vi "恢复参数.vi"(8 "仪器公式":T1(array[cluster]), 9 "量程参数":T2(array[cluster]), 10 "试剂容量参数":T3, 11 "外设参数":cluster{"外设配置":T4, "error out":errorcluster} {"外设配置"."阀方向" items=["顺时针", "逆时针", "就近"]; "外设配置"."总氮x公式0" items=["0", "1"]; "外设配置"."光谱仪类型" items=["1型", "2型", "3型", "2型氙灯联控"]; "外设配置"."泵阀量" items=["9通"=9, "10通"=10, "12通"=12]; "外设配置"."泵类型" items=["1型", "2型", "sy04型+旋转阀"]}) -> (3 "恢复结果":string)   [LabVIEW 2016, in "斯坦道氨氮.lvlib"]
uses:
  <vilib>/NI/Progress Bar/Progress Bar.lvlib
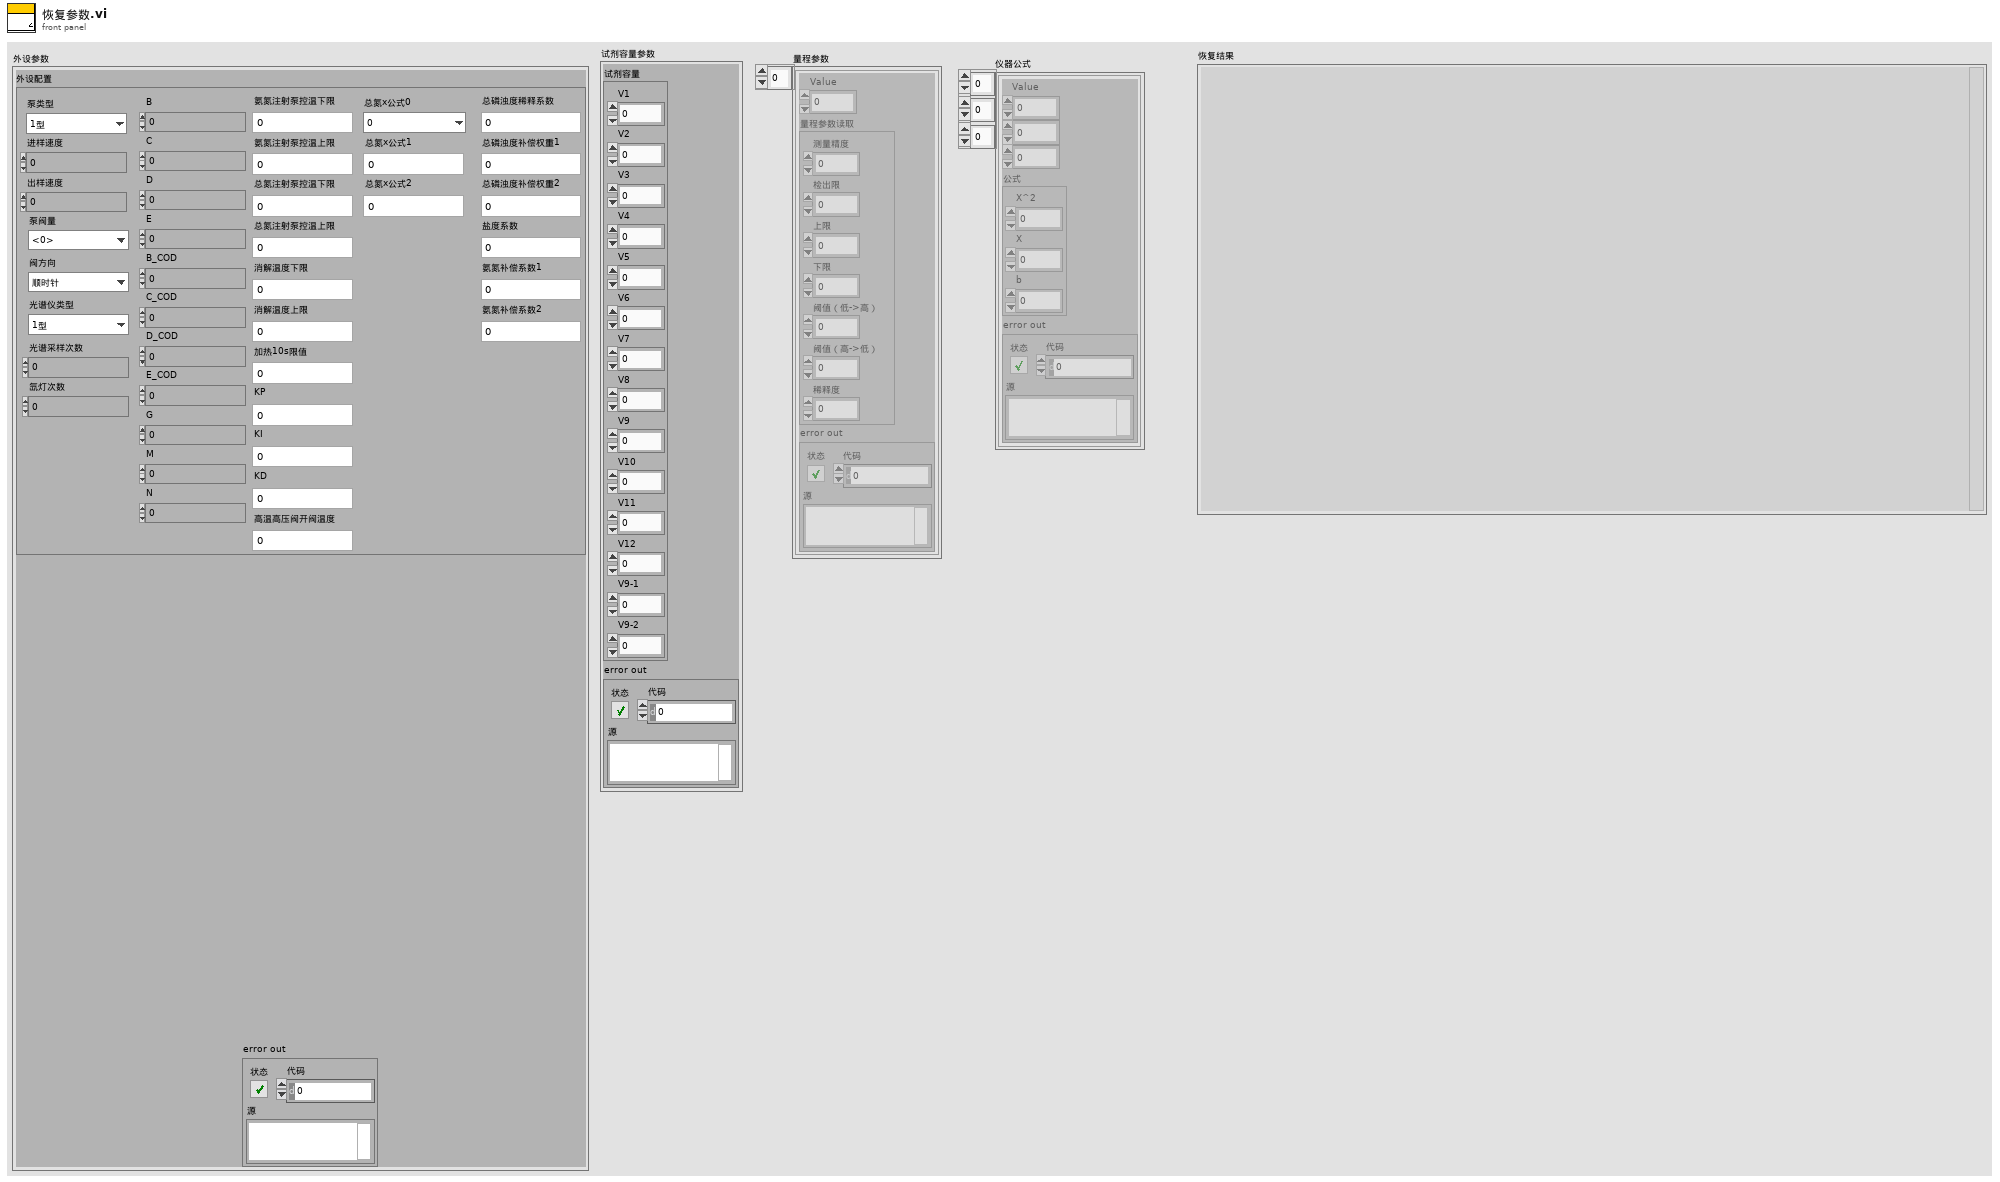
[diagram p1: front panel]
types:
  T1 = cluster{"Value":u16, i32, i32, "公式":cluster{"X^2":dbl, "X":dbl, "b":dbl}, "error out":errorcluster}[][][]
  T2 = cluster{"Value":u16, "量程参数读取":cluster{"测量精度":u16, "检出限":dbl, "上限":dbl, "下限":dbl, "阈值（低->高）":dbl, "阈值（高->低）":dbl, "稀释度":dbl}, "error out":errorcluster}[]
  T3 = cluster{"试剂容量":cluster{"V1":sgl, "V2":sgl, "V3":sgl, "V4":sgl, "V5":sgl, "V6":sgl, "V7":sgl, "V8":sgl, "V9":sgl, "V10":sgl, "V11":sgl, "V12":sgl, "V9-1":sgl, "V9-2":sgl}, "error out":errorcluster}
  T4 = typedef "斯坦道氨氮.lvlib/V3 A版外设参数.ctl" = cluster{"泵类型":u8, "进样速度":u32, "出样速度":u32, "泵阀量":u8, "阀方向":u8, "光谱仪类型":u8, "光谱采样次数":u8, "氙灯次数":u8, "B":u16, "C":u16, "D":u16, "E":u16, "B_COD":u16, "C_COD":u16, "D_COD":u16, "E_COD":u16, "G":u16, "M":u16, "N":u16, "氨氮注射泵控温下限":sgl, "氨氮注射泵控温上限":sgl, "总氮注射泵控温下限":sgl, "总氮注射泵控温上限":sgl, "消解温度下限":sgl, "消解温度上限":sgl, "加热10s限值":sgl, "KP":sgl, "KI":sgl, "KD":sgl, "高温高压阀开阀温度":sgl, "总氮x公式0":u8, "总氮x公式1":sgl, "总氮x公式2":sgl, "总磷浊度稀释系数":sgl, "总磷浊度补偿权重1":sgl, "总磷浊度补偿权重2":sgl, "盐度系数":sgl, "氨氮补偿系数1":sgl, "氨氮补偿系数2":sgl}
  T5 = enum16{"恢复外设参数", "恢复试剂容量参数", "恢复量程参数", "恢复仪器公式", "结束"}
  T6 = cluster{"V1":sgl, "V2":sgl, "V3":sgl, "V4":sgl, "V5":sgl, "V6":sgl, "V7":sgl, "V8":sgl, "V9":sgl, "V10":sgl, "V11":sgl, "V12":sgl, "V9-1":sgl, "V9-2":sgl}
  T7 = cluster{"测量精度":u16, "检出限":dbl, "上限":dbl, "下限":dbl, "阈值（低->高）":dbl, "阈值（高->低）":dbl, "稀释度":dbl}
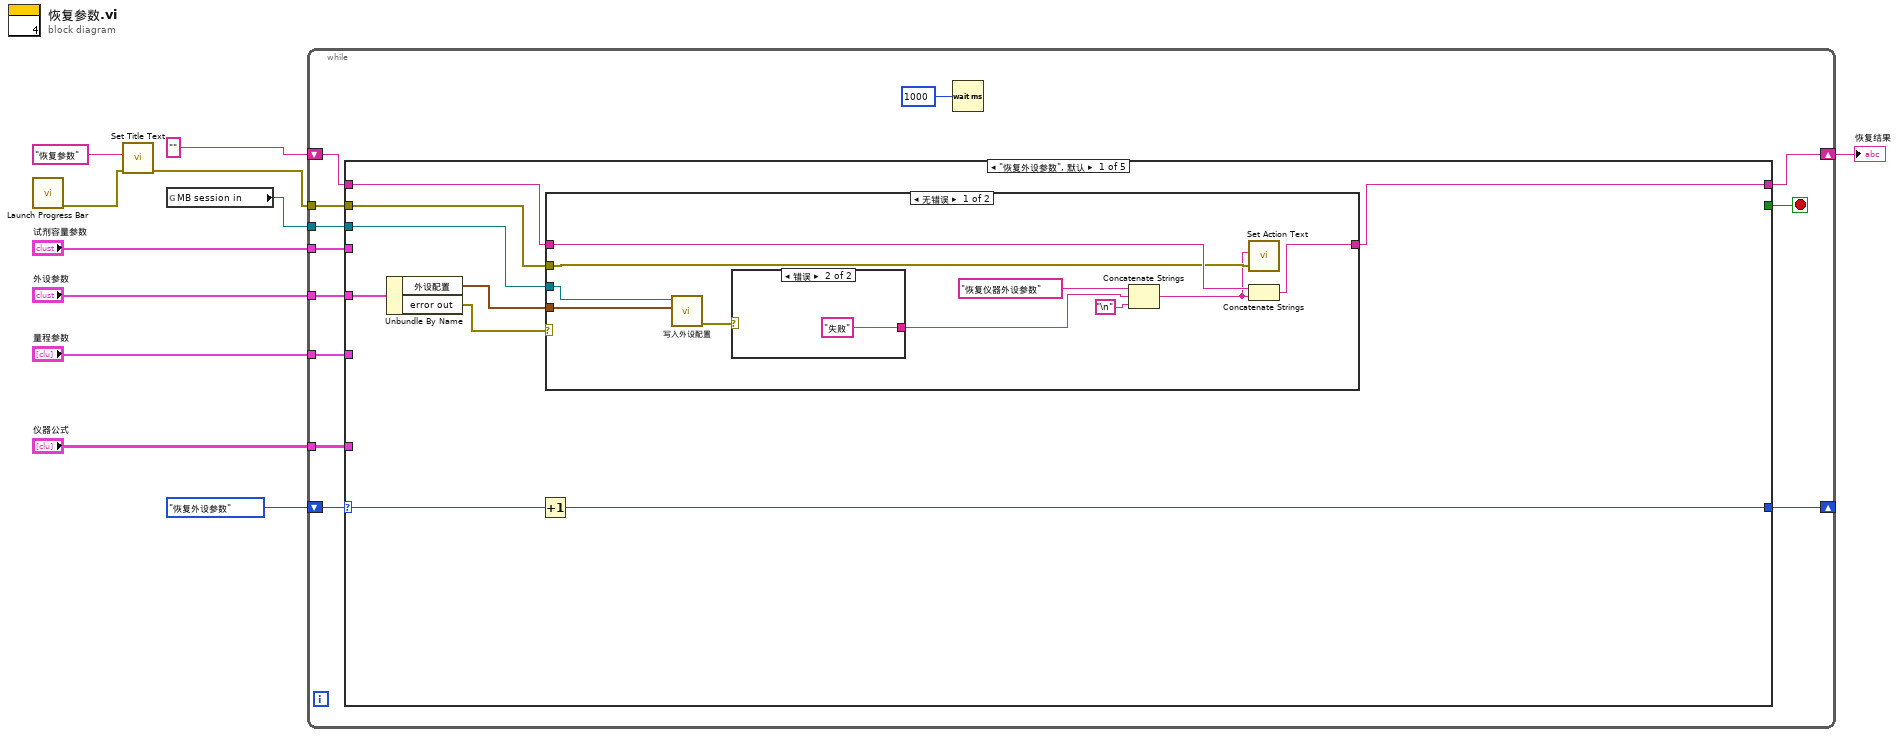
[diagram p0: block diagram]
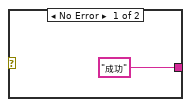
[diagram p2: hidden frame]
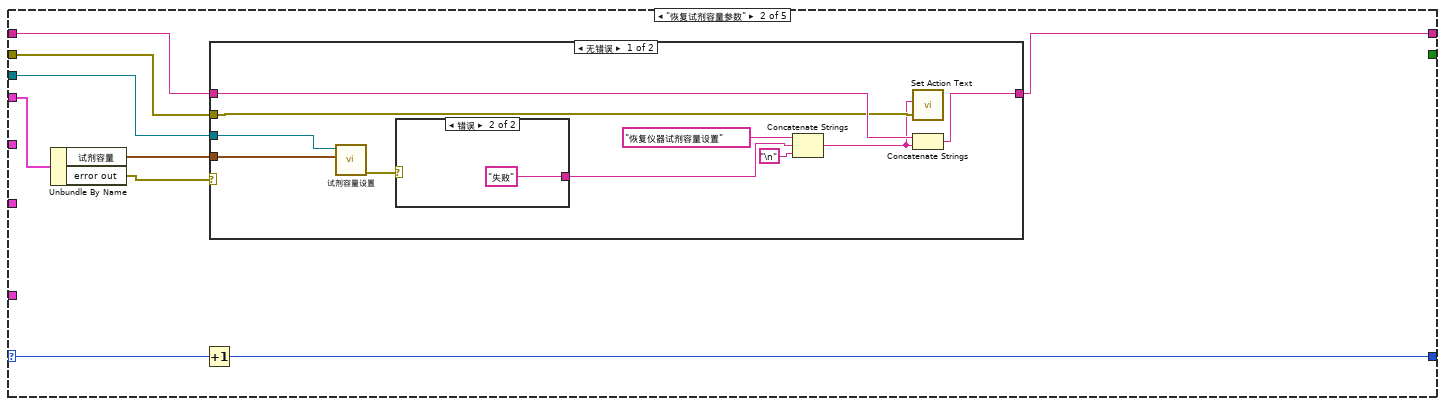
[diagram p4: hidden frame]
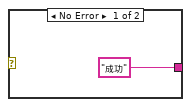
[diagram p5: hidden frame]
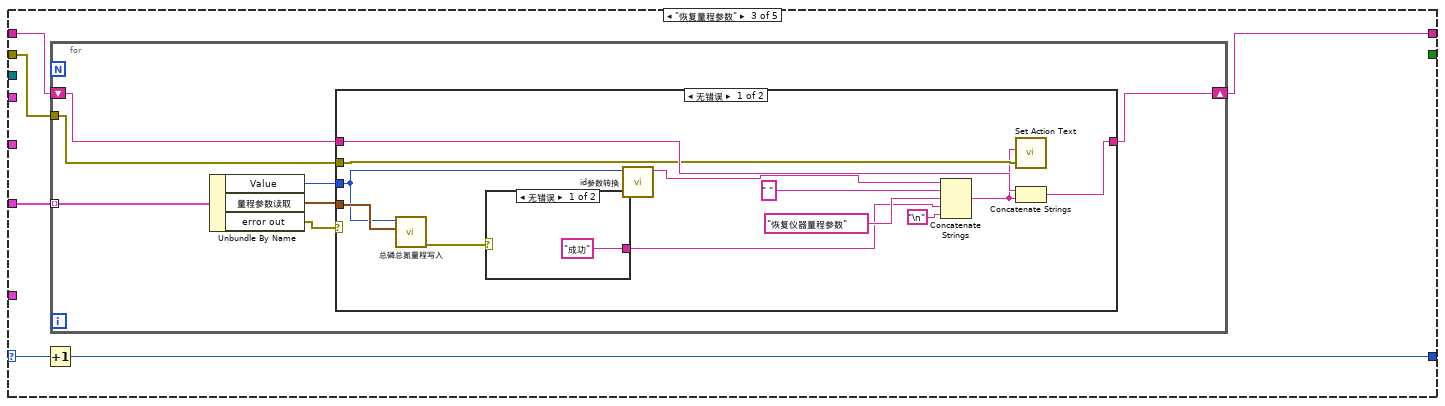
[diagram p7: hidden frame]
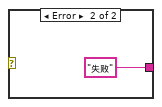
[diagram p8: hidden frame]
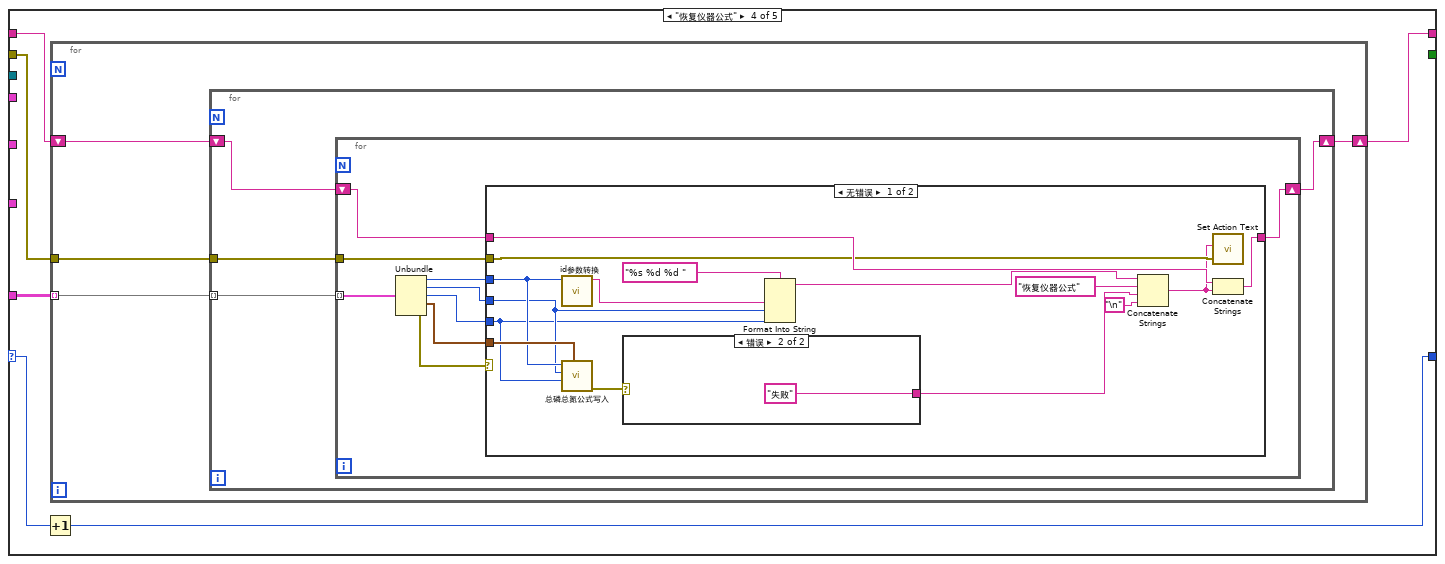
[diagram p10: hidden frame]
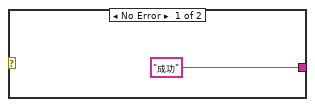
[diagram p11: hidden frame]
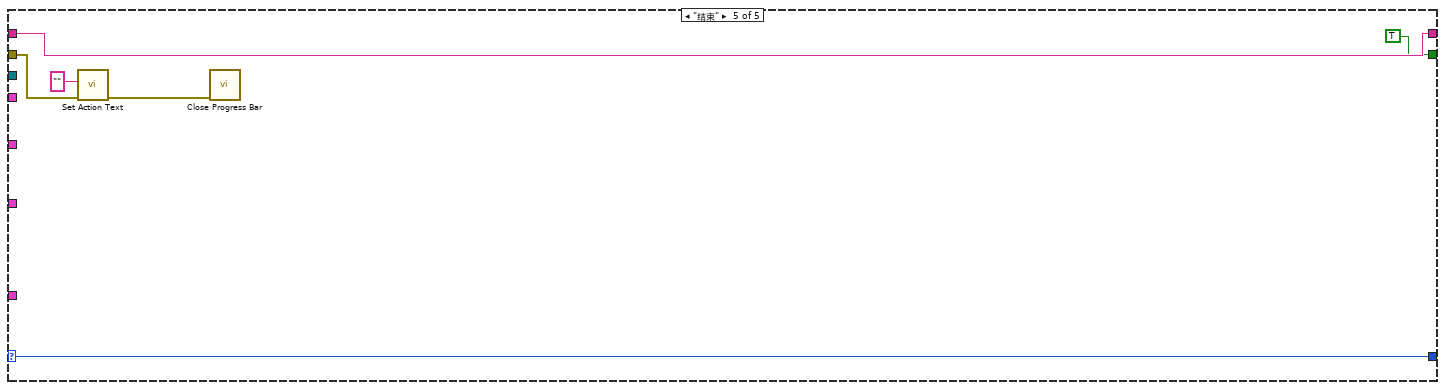
[diagram p13: hidden frame]
diagram:
  n1 = call <vilib>:"Launch Progress Bar.vi"() -> ("error out"=w3:errorcluster)  [unwired: 10 in, 1 out]
  n2 = call <vilib>:"Set Title Text.vi"("error in (no error)"=w3, "Installer Title"="恢复参数") -> ("error out"=w2:errorcluster)  [unwired: 9 in]
  n3 = global read "VAR总磷总氮全局变量.vi" "MB session in"() -> (w8:refnum<class "MB_Master.lvclass">)
  n4 = while {
    shift-right: [w22] -> _
    shift-left: T5."恢复外设参数" ("枚举") -> [w23]
    tunnel: "外设参数" -> [w21]
    shift-right: [w15] -> w4
    shift-left: "" -> [w20]
    tunnel: w8 -> [w19]
    tunnel: "试剂容量参数" -> [w18]
    tunnel: "量程参数" -> [w17]
    tunnel: "仪器公式" -> [w16]
    tunnel: w2 -> [w13]
    stop <- w14 stop-if-true
    n5 = case shown="\"恢复外设参数\", 默认" w23 {
      selector: w23 -> [w32 w54 w73 w101 w142]
      tunnel: [w31 w53 w72 w100 w142] -> w22
      tunnel: w21 -> [w30 _ _ _ _]
      tunnel: w20 -> [w27 w48 w70 w98 w141]
      tunnel: w19 -> [w26 w50 _ _ _]
      tunnel: w18 -> [_ w52 _ _ _]
      tunnel: w17 -> [_ _ w71 _ _]
      tunnel: w16 -> [_ _ _ w99 _]
      tunnel: [w25 w47 w69 w97 w141] -> w15
      tunnel: [_ _ _ _ TRUE] -> w14
      tunnel: w13 -> [w24 w46 w68 w96 w139]
      frame "恢复外设参数", Default {
        n6 = Unbundle By Name(w30) -> ("外设配置"=w29:T4, "error out"=w28:errorcluster)
        n7 = Increment(x=w32) -> (x+1=w31:T5)
        n8 = case shown="无错误" w28 {
          tunnel: w26 -> [w42 _]
          tunnel: w29 -> [w41 _]
          tunnel: [w35 w45] -> w25
          tunnel: w27 -> [w36 w45]
          tunnel: w24 -> [w34 _]
          frame No Error {
            n9 = call "写入外设配置.vi"("外设配置"=w41, "MB session in"=w42) -> ("error out"=w38:errorcluster)  [unwired: 8 in, 1 out]
            n10 = case shown="错误" w38 {
              tunnel: ["成功" "失败"] -> w39
              frame No Error {
              }
              frame Error {
              }
            }
            n11 = Concatenate Strings("恢复仪器外设参数" ("字符串"), w39, "\n") -> (w33:string)
            n12 = call <vilib>:"Set Action Text.vi"("error in (no error)"=w34, "Action Text"=w33) -> ()  [unwired: 9 in, 1 out]
            n13 = Concatenate Strings(w36, w33) -> (w35:string)
          }
          frame Error {
          }
        }
      }
      frame "恢复试剂容量参数" {
        n14 = Unbundle By Name(w52) -> ("试剂容量"=w51:T6, "error out"=w49:errorcluster)
        n15 = Increment(x=w54) -> (x+1=w53:T5)
        n16 = case shown="无错误" w49 {
          tunnel: w51 -> [w64 _]
          tunnel: w50 -> [w63 _]
          tunnel: w48 -> [w58 w67]
          tunnel: [w57 w67] -> w47
          tunnel: w46 -> [w56 _]
          frame No Error {
            n17 = call "试剂容量设置.vi"("试剂容量"=w64, "MB session in"=w63) -> ("error out"=w60:errorcluster)  [unwired: 8 in, 1 out]
            n18 = case shown="错误" w60 {
              tunnel: ["成功" "失败"] -> w61
              frame No Error {
              }
              frame Error {
              }
            }
            n19 = Concatenate Strings("恢复仪器试剂容量设置" ("字符串"), w61, "\n") -> (w55:string)
            n20 = call <vilib>:"Set Action Text.vi"("error in (no error)"=w56, "Action Text"=w55) -> ()  [unwired: 9 in, 1 out]
            n21 = Concatenate Strings(w58, w55) -> (w57:string)
          }
          frame Error {
          }
        }
      }
      frame "恢复量程参数" {
        n22 = Increment(x=w73) -> (x+1=w72:T5)
        n23 = for {
          tunnel: w71 -> [w80] mode=indexing
          shift-right: [w75] -> w69
          shift-left: w70 -> [w76]
          tunnel: w68 -> [w74]
          n24 = Unbundle By Name(w80) -> ("Value"=w78:u16, "量程参数读取"=w79:T7, "error out"=w77:errorcluster)
          n25 = case shown="无错误" w77 {
            tunnel: w79 -> [w92 _]
            tunnel: w78 -> [w88 _]
            tunnel: w76 -> [w84 w95]
            tunnel: [w83 w95] -> w75
            tunnel: w74 -> [w82 _]
            frame No Error {
              n26 = call "总磷总氮量程写入.vi"("量程参数写入"=w92, "测量参数"=w88) -> ("error out"=w89:errorcluster)  [unwired: 8 in]
              n27 = case shown="无错误" w89 {
                tunnel: ["成功" "失败"] -> w90
                frame No Error {
                }
                frame Error {
                }
              }
              n28 = call "id参数转换.vi"("id"=w88) -> ("table输出"=w87:string)  [unwired: 9 in, 1 out]
              n29 = Concatenate Strings(w87, " " ("字符串"), "恢复仪器量程参数" ("字符串"), w90, "\n") -> (w81:string)
              n30 = call <vilib>:"Set Action Text.vi"("error in (no error)"=w82, "Action Text"=w81) -> ()  [unwired: 9 in, 1 out]
              n31 = Concatenate Strings(w84, w81) -> (w83:string)
            }
            frame Error {
            }
          }
        }
      }
      frame "恢复仪器公式" {
        n32 = Increment(x=w101) -> (x+1=w100:T5)
        n33 = for {
          tunnel: w99 -> [w105] mode=indexing
          shift-right: [w103] -> w97
          shift-left: w98 -> [w104]
          tunnel: w96 -> [w102]
          n34 = for {
            tunnel: w105 -> [w109] mode=indexing
            shift-right: [w107] -> w103
            shift-left: w104 -> [w108]
            tunnel: w102 -> [w106]
            n35 = for {
              tunnel: w109 -> [w118] mode=indexing
              shift-right: [w111] -> w107
              shift-left: w108 -> [w112]
              tunnel: w106 -> [w110]
              n36 = Unbundle(w118) -> ("Value"=w116:u16, w115:i32, w114:i32, "公式"=w113:cluster{"X^2":dbl, "X":dbl, "b":dbl}, "error out"=w117:errorcluster)
              n37 = case shown="无错误" w117 {
                tunnel: w116 -> [w126 _]
                tunnel: w115 -> [w125 _]
                tunnel: w114 -> [w124 _]
                tunnel: w113 -> [w133 _]
                tunnel: w112 -> [w122 w136]
                tunnel: [w121 w136] -> w111
                tunnel: w110 -> [w120 _]
                frame No Error {
                  n38 = call "id参数转换.vi"("id"=w126) -> ("table输出"=w129:string)  [unwired: 9 in, 1 out]
                  n39 = call "总磷总氮公式写入.vi"("公式"=w133, "量程"=w124, "测量模式"=w125, "测量参数"=w126) -> ("error out"=w127:errorcluster)  [unwired: 7 in]
                  n40 = case shown="错误" w127 {
                    tunnel: ["成功" "失败"] -> w132
                    frame No Error {
                    }
                    frame Error {
                    }
                  }
                  n41 = Format Into String(format string="%s %d %d " ("格式字符串"), w129, w125, w124) -> (resulting string=w128:string)  [unwired: 2 in, 1 out]
                  n42 = Concatenate Strings(w128, "恢复仪器公式" ("字符串"), w132, "\n") -> (w119:string)
                  n43 = call <vilib>:"Set Action Text.vi"("error in (no error)"=w120, "Action Text"=w119) -> ()  [unwired: 9 in, 1 out]
                  n44 = Concatenate Strings(w122, w119) -> (w121:string)
                }
                frame Error {
                }
              }
            }
          }
        }
      }
      frame "结束" {
        n45 = call <vilib>:"Set Action Text.vi"("error in (no error)"=w139, "Action Text"="") -> ("error out"=w138:errorcluster)  [unwired: 9 in]
        n46 = call <vilib>:"Close Progress Bar.vi"("error in (no error)"=w138) -> ()  [unwired: 9 in, 2 out]
      }
    }
    n47 = Wait (ms)(milliseconds to wait=u32 1000 ("等待时间（毫秒）")) -> ()  [unwired: 1 out]
  }
  "恢复结果" <- w4
